vi "Initialization File Parser.vi"(8 "error in (no error)":errorcluster, 11 "default init file name":string="P350 Experiment Init A") -> (0 "error out":errorcluster, 1 "Timing Control Parameters":T1={"N cycles for averaging"=300, "N points per measurement"=1000, "Measurment time interval"=2e-05} {"Measurment time interval" format="%.2e"}, 2 "Temperature Control Parameters":T2={"Start Temp"=40.0, "Temp Step"=10.0, "End Temp"=60.0} {"End Temp" format="%.2f"; "Temp Step" format="%.2f"; "Start Temp" format="%.2f"}, 3 "file path used":path, 5 "Auto Launch Data Viewer at End":bool)   [LabVIEW 2014]
doc: "This vi parses out control information from a initialization file. It is used in the P350 C(T) experiment.\n\nPaul K Dixon\nPhysics 350\nCSUSB Physics"
panel:
  # "Physics 350\nPaul K Dixon\nInitialization File Parser"
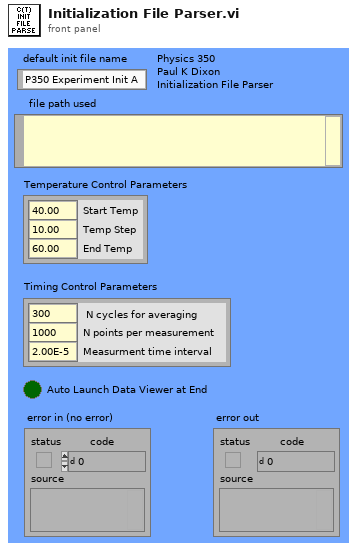
[diagram p1: front panel]
types:
  T1 = cluster{"N cycles for averaging":i32, "N points per measurement":i32, "Measurment time interval":dbl}
  T2 = cluster{"Start Temp":dbl, "Temp Step":dbl, "End Temp":dbl}
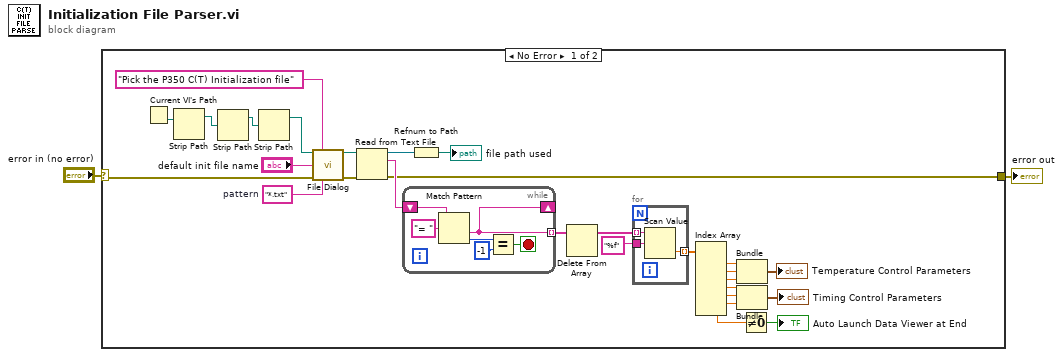
[diagram p0: block diagram]
diagram:
  n1 = case shown="No Error" "error in (no error)" {
    selector: "error in (no error)" -> [w9 w40]
    tunnel: [w10 w40] -> w1
    frame No Error {
      w3 = "*.txt"  # pattern
      n2 = Current VI's Path() -> (path=w16:path)
      n3 = Strip Path(path=w16) -> (stripped path=w15:path)  [unwired: 1 out]
      n4 = Strip Path(path=w15) -> (stripped path=w14:path)  [unwired: 1 out]
      n5 = Strip Path(path=w14) -> (stripped path=w8:path)  [unwired: 1 out]
      n6 = call "File Dialog"("start path"=w8, "prompt"="Pick the P350 C(T) Initialization file", "default name"="default init file name", "error in"=w9, "pattern (all files)"=w3) -> ("selected path"=w6:path, "error out"=w7:errorcluster)  [unwired: 7 in, 2 out]
      n7 = Read from Text File(file (use dialog)=w6, error in=w7) -> (refnum out=w12:refnum<file>, text=w13:string, error out=w10:errorcluster)  [unwired: 3 out]
      n8 = while {
        tunnel: [w31] -> w30 mode=indexing
        shift-left: w13 -> [w35]
        shift-right: [w31] -> _
        stop <- w32 stop-if-true
        n9 = Match Pattern(string=w35, regular expression="= ") -> (after substring=w31:string, offset past match=w34:i32)  [unwired: 3 out]
        n10 = Equal?(x=w34, y=-1) -> (x = y?=w32:bool)
      }
      n11 = Refnum to Path(1:w12) -> (0:→"file path used":path)
      n12 = Delete From Array(array=w30) -> (array with subset deleted=w29:string[])  [unwired: 2 in, 1 out]
      n13 = for {
        tunnel: w29 -> [w39] mode=indexing
        tunnel: "%f" ("format string") -> [w38]
        tunnel: [w37] -> w27 mode=indexing
        n14 = Scan Value(string=w39, format string=w38) -> (value=w37:dbl)  [unwired: 2 out]
      }
      n15 = Index Array(array=w27) -> (element #1=w24:dbl, element #2=w23:dbl, element #3=w22:dbl, element #4=w20:dbl, element #5=w19:dbl, element #6=w18:dbl, element #7=w26:dbl)  [unwired: 7 in]
      n16 = Bundle(w24, w23, w22) -> (→"Temperature Control Parameters":cluster{dbl, dbl, dbl})  [unwired: 1 out]
      n17 = Bundle(w20, w19, w18) -> (→"Timing Control Parameters":cluster{dbl, dbl, dbl})  [unwired: 1 out]
      n18 = Not Equal To 0?(x=w26) -> (x != 0?=→"Auto Launch Data Viewer at End":bool)
    }
    frame Error {
    }
  }
  "error out" <- w1
